vi "In Bounds 1D.vi"(0 "Top":T1 {"Axial Force" format="%.4f"; "Lateral Force" format="%.4f"}, 1 "Bottom":T1 {"Axial Force" format="%.4f"; "Lateral Force" format="%.4f"}, 4 "Axial":dbl) -> (14 "InBounds":bool)   [LabVIEW 2016]
uses:
  Typedefs/ForcePair.ctl
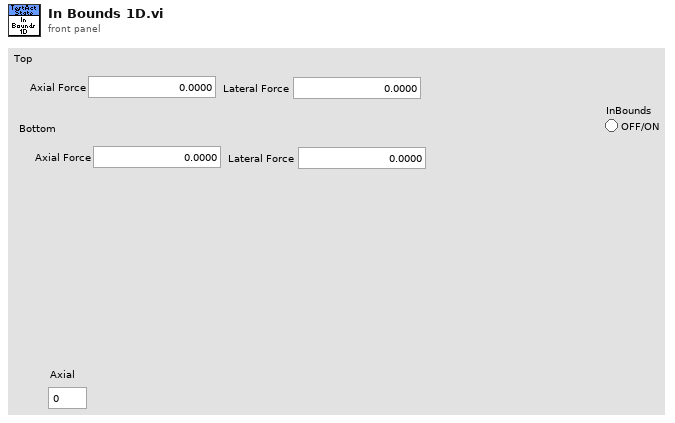
[diagram p1: front panel]
types:
  T1 = typedef "ForcePair.ctl" = cluster{"Axial Force":dbl, "Lateral Force":dbl}
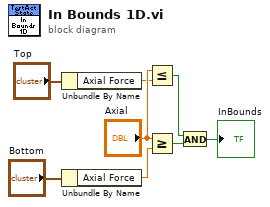
[diagram p0: block diagram]
diagram:
  n1 = Unbundle By Name("Top") -> ("Axial Force"=w5:dbl)
  n2 = Unbundle By Name("Bottom") -> ("Axial Force"=w4:dbl)
  n3 = Less Or Equal?(x="Axial", y=w5) -> (x <= y?=w3:bool)
  n4 = Greater Or Equal?(x="Axial", y=w4) -> (x >= y?=w2:bool)
  n5 = And(x=w3, y=w2) -> (x .and. y?=→"InBounds":bool)
